vi "test - Set VI Icon Colour - Orange.vi"(8 "error in (no error)":errorcluster, 11 "TestCase in":refnum<class "Create New Assert Tester.lvclass">) -> (0 "error out":errorcluster, 3 "TestCase out":refnum<class "Create New Assert Tester.lvclass">)   [LabVIEW 2018, in "Create New Assert Tester.lvclass"]
uses:
  Create New Assert Tester.lvclass
  <vilib>/picture/picture.llb/imagedata.ctl
  <vilib>/addons/_JKI Toolkits/VI Tester/TestCase.llb/TestCase.lvclass
  Plugins/Utility/Set VI Icon Colour.vi
  C:/Program Files (x86)/National Instruments/LabVIEW 2018/vi.lib/addons/_JKI Toolkits/VI Tester/TestCase.llb/TestCase.lvclass
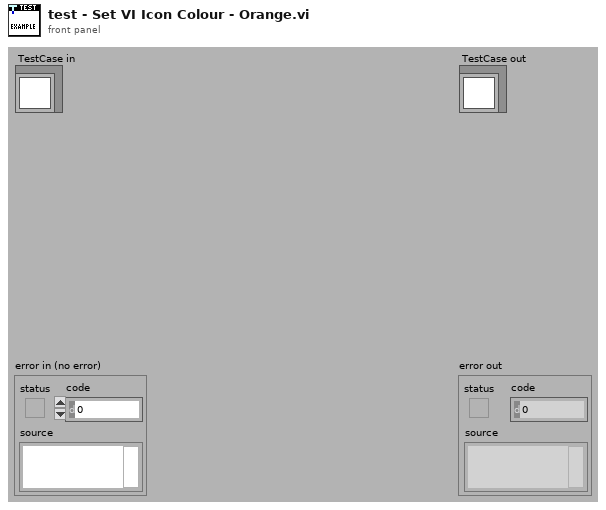
[diagram p1: front panel]
types:
  T1 = typedef "imagedata.ctl" = cluster{"image type":i32, "image depth":i32, "image":u8[], "mask":u8[], "colors":u32[], "Rectangle":cluster{"left":i16, "top":i16, "right":i16, "bottom":i16}}
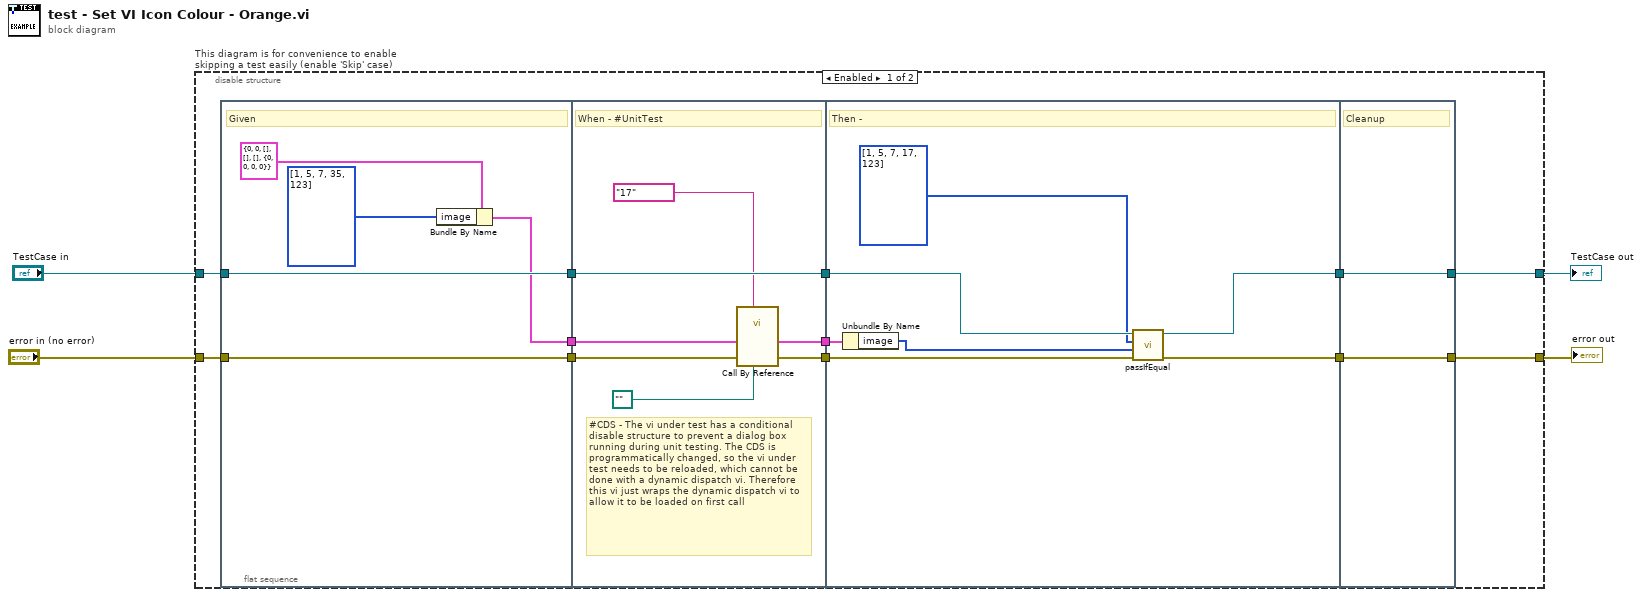
[diagram p0: block diagram]
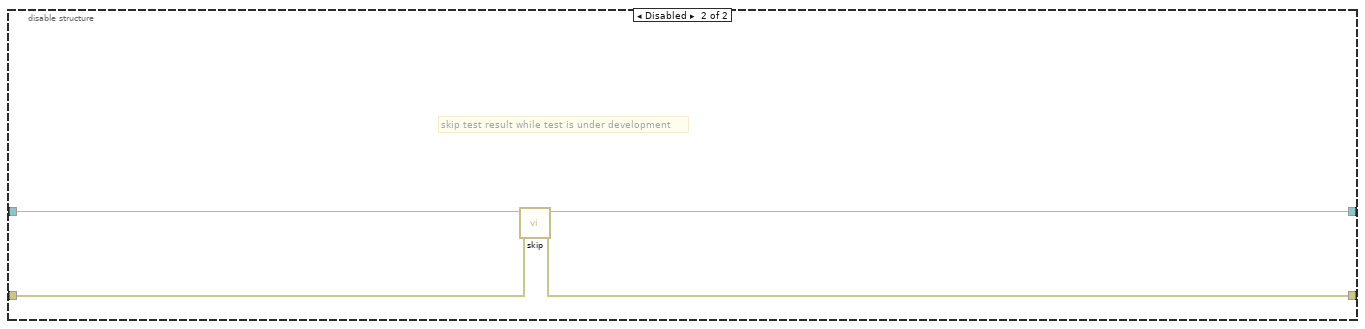
[diagram p2: hidden frame]
diagram:
  n1 = disable-structure "This diagram is for convenience to enable skipping a test easily (enable 'Skip' case)" shown="Enabled" {
    disable-tunnel: "TestCase in" -> [w10 w41]
    disable-tunnel: [w7 w39] -> w1
    disable-tunnel: [w8 w40] -> w3
    disable-tunnel: "error in (no error)" -> [w9 w38]
    frame Enabled {
      n2 = flat-sequence {
        tunnel: w9 -> [w20]
        tunnel: w10 -> [w21]
        tunnel: [w21] -> w16
        tunnel: [w20] -> w15
        tunnel: [w18] -> w5
        tunnel: [w28] -> w14
        tunnel: [w26] -> w13
        tunnel: w16 -> [w28]
        tunnel: w15 -> [w27]
        tunnel: [w25] -> w6
        tunnel: w5 -> [w23]
        tunnel: [w32] -> w12
        tunnel: [w34] -> w11
        tunnel: w14 -> [w33]
        tunnel: w13 -> [w35]
        tunnel: w6 -> [w31]
        tunnel: [w36] -> w8
        tunnel: [w37] -> w7
        tunnel: w12 -> [w37]
        tunnel: w11 -> [w36]
        frame #0 {
          # "Given"
          n3 = Bundle By Name(cluster=T1 {"image type"=0, "image depth"=0, "image"=[], "mask"=[], "colors"=[], "Rectangle"={"left"=0, "top"=0, "right"=0, "bottom"=0}} ("ImageData (Test IP only)"), "image"=u8[] [1, 5, 7, 35, 123]) -> (w18:T1)
        }
        frame #1 {
          # "#CDS - The vi under test has a conditional disable structure to prevent a dialog box running during unit testing. The CDS is programmatically changed, so the vi under test needs to be reloaded, which cannot be done with a dynamic dispatch vi. Therefore this vi just wraps the dynamic dispatch vi to allow it to be loaded on first call"
          # "When - #UnitTest"
          n4 = call-by-ref "?"("VI Path"=path "", "Colour string"="17" ("Type"), "error in (no error)"=w27, "ImageData (Test IP only)"=w23) -> ("error out"=w26:errorcluster, "ImageData (Test OP only)"=w25:T1)  [unwired: 8 in, 2 out]
        }
        frame #2 {
          # "Then -"
          n5 = Unbundle By Name(w31) -> ("image"=w30:u8[])
          n6 = call-dynamic "passIfEqual.vi"("error in (no error)"=w35, "y"=w30, "x"=u8[] [1, 5, 7, 17, 123] ("image"), "TestCase in"=w33) -> ("error out"=w34:errorcluster, "TestCase out"=w32:refnum<class "Create New Assert Tester.lvclass">)  [unwired: 6 in]
        }
        frame #3 {
          # "Cleanup"
        }
      }
    }
    frame Disabled {
      # "skip test result while test is under development"
      n7 = call <vilib>:"skip.vi"("error in (no error)"=w38, "TestCase in"=w41) -> ("error out"=w40:errorcluster, "TestCase out"=w39:refnum<class "Create New Assert Tester.lvclass">)  [unwired: 8 in]
    }
  }
  "error out" <- w3
  "TestCase out" <- w1
